vi "Get Engine Update.vi"(8 "Error In":errorcluster, 11 "ECU COM Port":refnum<visa-resource-name>) -> (0 "Error Out":errorcluster, 1 "Temperature":string, 2 "RPMs":string, 3 "ECU COM Port Out":refnum<visa-resource-name>)   [LabVIEW 2017]
doc: "<b>Description</b>\nThis VI gets an update of RPM and Temperature from the engine.\n\n<b>Inputs</b>\nECU COM Port: The com port of the ECU.\n\n<b>Outputs</b>\nECU COM Port Out: The com port of the ECU.\nRPMs: The measured RPMs from the engine.\nTemperature: The measured temperature from the engine."
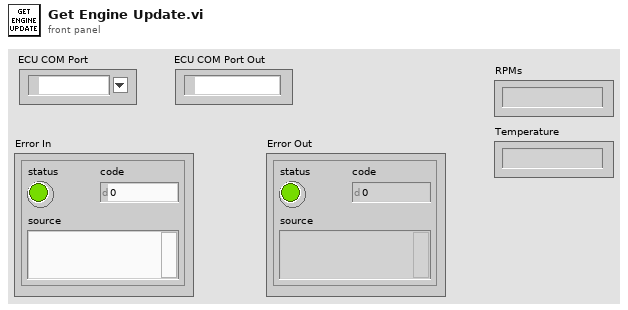
[diagram p1: front panel]
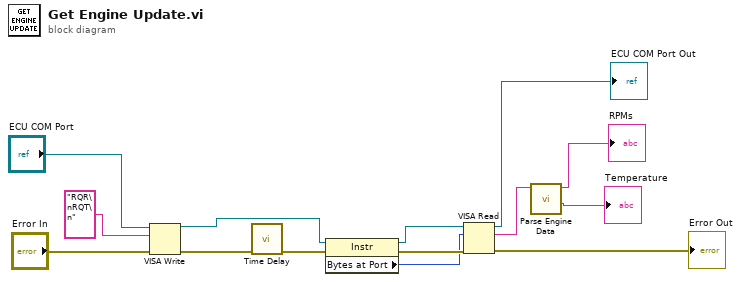
[diagram p0: block diagram]
diagram:
  n1 = VISA Write(VISA resource name="ECU COM Port", write buffer="RQR\nRQT\n", error in (no error)="Error In") -> (VISA resource name out=w7:refnum<visa-resource-name>, error out=w11:errorcluster)  [unwired: 1 out]
  n2 = call "Time Delay"("error in (no error)"=w11) -> ("error out"=w10:errorcluster)  [unwired: 10 in]
  n3 = property class="Instr"(reference=w7, error in=w10) -> (reference out=w8:refnum<visa-resource-name>, error out=w9:errorcluster, "Bytes at Port"=w6:u32)
  n4 = VISA Read(VISA resource name=w8, byte count=w6, error in (no error)=w9) -> (VISA resource name out=→"ECU COM Port Out":refnum<visa-resource-name>, read buffer=w4:string, error out=→"Error Out":errorcluster)  [unwired: 1 out]
  n5 = call "Parse Engine Data.vi"("Input"=w4) -> ("Temperature"=→"Temperature":string, "RPMs"=→"RPMs":string)  [unwired: 9 in]
